vi "Write XLSX.vi"(8 "error in (no error)":errorcluster, 9 "stream":refnum<k24>, 11 "XSSFWorkbook Reference":refnum<k24>) -> (0 "error out":errorcluster, 3 "XSSFWorkbook Reference out":refnum<k24>)   [LabVIEW 2013]
uses:
  C:/PhaeronGit/LVNPOI/Resources/NPOI 2.1.1 dotnet4/NPOI.OOXML.dll
  Resources/NPOI 2.1.1 dotnet4/NPOI.OOXML.dll
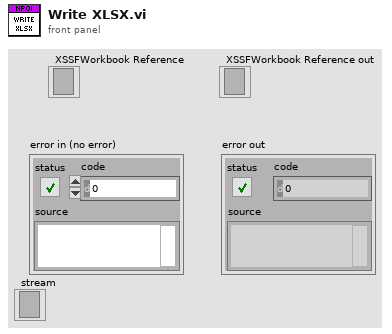
[diagram p1: front panel]
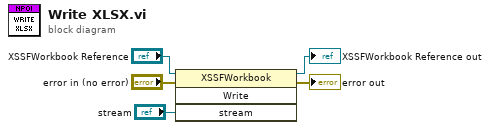
[diagram p0: block diagram]
diagram:
  n1 = invoke class="XSSFWorkbook" method="Write"(reference="XSSFWorkbook Reference", error in="error in (no error)", "stream"="stream") -> (reference out=→"XSSFWorkbook Reference out":refnum<k24>, error out=→"error out":errorcluster)  [unwired: 1 in, 2 out]
